vi "ConvertTextBasedCodeToLabVIEW_MakenamesBetter.vi"(11 "ClassesIn":T1[](array[typedef])) -> (3 "ClassesOut":T1[](array[typedef]))   [LabVIEW 2014]
uses:
  <resource>/Framework/Providers/Open_GDS/ClassProviders/Common/String/GDSString_ClassDescriptionType.ctl
  <resource>/Framework/Providers/Open_GDS/ClassProviders/Common/String/GDSString_AccessScopeModifierType.ctl
  <resource>/Framework/Providers/Open_GDS/ClassProviders/Common/String/GDSString_ModifierType.ctl
  <resource>/Framework/Providers/Open_GDS/ClassProviders/Common/String/GDSString_MethodDescriptionType.ctl
  <resource>/Framework/Providers/Open_GDS/ClassProviders/Common/CommonVIs/CommonVIs_AttributeType.ctl
  <resource>/Framework/Providers/Open_GDS/ClassProviders/Common/CommonVIs/CommonVIs_AttributeDataType.ctl
  <resource>/Framework/Providers/Open_GDS/ClassProviders/Common/CommonVIs/CommonVIs_PropertyType.ctl
  <resource>/Framework/Providers/Open_GDS/ClassProviders/Common/String/GDSString_ClassParentType.ctl
  <resource>/Framework/Providers/Open_GDS/ClassProviders/Common/String/GDSString_ClassType.ctl
  <resource>/Framework/Providers/Open_GDS/ClassProviders/Common/String/GDSString_ClassOwnerType.ctl
  <resource>/Framework/Providers/Open_GDS/ClassProviders/Common/CommonVIs/CommonVIs_EnumType.ctl
  <resource>/Framework/Providers/Open_GDS/ClassProviders/Common/CommonVIs/CommonVIs_StructType.ctl
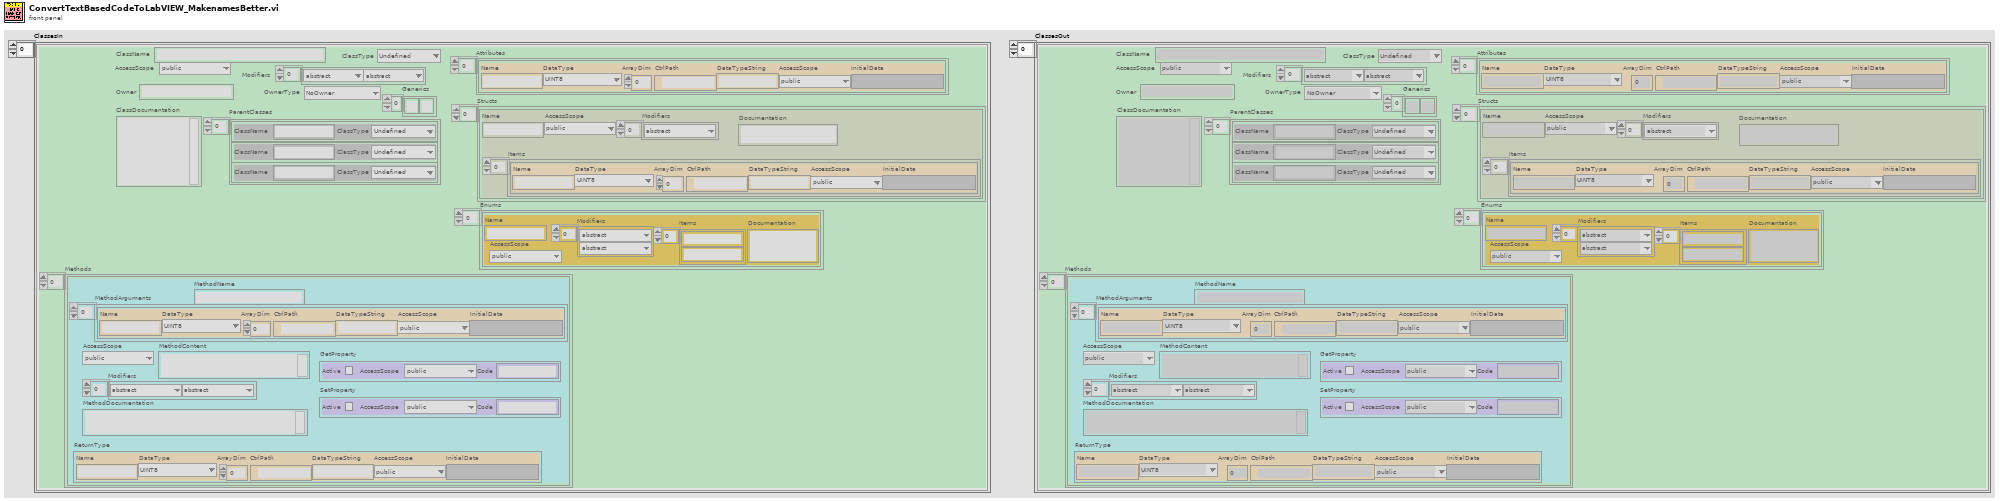
[diagram p1: front panel]
types:
  T1 = typedef "GDSString_ClassDescriptionType.ctl" = cluster{"ClassName":string, "AccessScope":T2, "Modifiers":T3[], "ClassDocumentation":string, "Methods":T4[], "ParentClasses":T8[], "ClassType":T9, "Owner":string, "OwnerType":T10, "Generics":string[], "Attributes":T5[], "Enums":T11[], "Structs":T12[]}
  T2 = typedef "GDSString_AccessScopeModifierType.ctl" = enum16{"public", "private", "protected", "internal"}
  T3 = typedef "GDSString_ModifierType.ctl" = enum16{"abstract", "static", "final", "synchronized", "strictfp", "async", "const", "event", "extern", "new", "native ", "override", "partial", "readonly", "sealed", "unsafe", "virtual", "volatile"}
  T4 = typedef "GDSString_MethodDescriptionType.ctl" = cluster{"ReturnType":T5, "MethodName":string, "AccessScope":T2, "Modifiers":T3[], "MethodDocumentation":string, "MethodContent":string, "MethodArguments":T5[], "GetProperty":T7, "SetProperty":T7}
  T5 = typedef "CommonVIs_AttributeType.ctl" = cluster{"Name":string, "DataType":T6, "ArrayDim":i32, "CtrlPath":path, "DataTypeString":string, "AccessScope":T2, "InitialData":variant}
  T6 = typedef "CommonVIs_AttributeDataType.ctl" = enum16{"UINT8", "INT8", "UINT16", "INT16", "UINT32", "INT32", "UINT64", "INT64", "SGL", "DBL", "EXT", "CSG", "CDB", "CXT", "TimeStamp", "STRING", "PATH", "BOOL", "ENUM", "RefNum", "VIRefNum", "LabVIEW Class", "Cluster", "Variant", "TypeDef", "Waveform", "LabVIEW Object", "Other", "void"}
  T7 = typedef "CommonVIs_PropertyType.ctl" = cluster{"Active":bool, "AccessScope":T2, "Code":string}
  T8 = typedef "GDSString_ClassParentType.ctl" = cluster{"ClassName":string, "ClassType":T9}
  T9 = typedef "GDSString_ClassType.ctl" = enum16{"Undefined", "Class", "Interface"}
  T10 = typedef "GDSString_ClassOwnerType.ctl" = enum16{"NoOwner", "Class", "Package/NameSpace"}
  T11 = typedef "CommonVIs_EnumType.ctl" = cluster{"Name":string, "AccessScope":T2, "Modifiers":T3[], "Items":string[], "Documentation":string}
  T12 = typedef "CommonVIs_StructType.ctl" = cluster{"Name":string, "AccessScope":T2, "Modifiers":T3[], "Items":T5[], "Documentation":string}
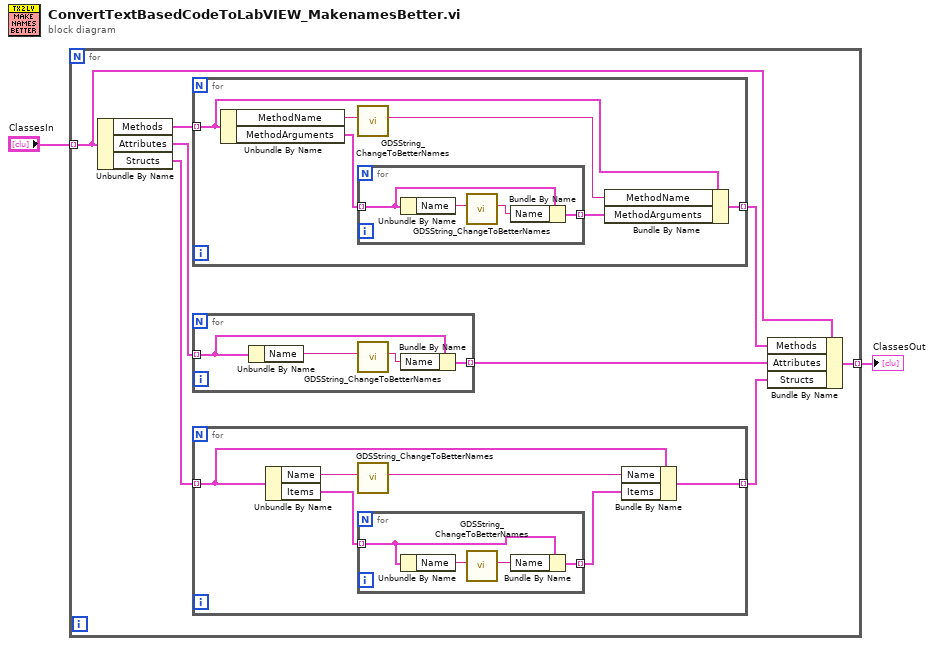
[diagram p0: block diagram]
diagram:
  n1 = for {
    tunnel: "ClassesIn" -> [w8] mode=indexing
    tunnel: [w3] -> w1 mode=indexing
    n2 = Unbundle By Name(w8) -> ("Methods"=w10:T4[], "Attributes"=w9:T5[], "Structs"=w5:T12[])
    n3 = for {
      tunnel: w10 -> [w29] mode=indexing
      tunnel: [w25] -> w7 mode=indexing
      n4 = Unbundle By Name(w29) -> ("MethodName"=w27:string, "MethodArguments"=w30:T5[])
      n5 = call <resource>:"GDSString_ChangeToBetterNames.vi"("NameIn"=w27) -> ("NameOut"=w26:string)  [unwired: 9 in, 1 out]
      n6 = for {
        tunnel: w30 -> [w33] mode=indexing
        tunnel: [w31] -> w28 mode=indexing
        n7 = Unbundle By Name(w33) -> ("Name"=w34:string)
        n8 = call <resource>:"GDSString_ChangeToBetterNames.vi"("NameIn"=w34) -> ("NameOut"=w32:string)  [unwired: 9 in, 1 out]
        n9 = Bundle By Name(cluster=w33, "Name"=w32) -> (w31:T5)
      }
      n10 = Bundle By Name(cluster=w29, "MethodName"=w26, "MethodArguments"=w28) -> (w25:T4)
    }
    n11 = for {
      tunnel: w9 -> [w23] mode=indexing
      tunnel: [w21] -> w6 mode=indexing
      n12 = Unbundle By Name(w23) -> ("Name"=w24:string)
      n13 = call <resource>:"GDSString_ChangeToBetterNames.vi"("NameIn"=w24) -> ("NameOut"=w22:string)  [unwired: 9 in, 1 out]
      n14 = Bundle By Name(cluster=w23, "Name"=w22) -> (w21:T5)
    }
    n15 = for {
      tunnel: w5 -> [w15] mode=indexing
      tunnel: [w11] -> w4 mode=indexing
      n16 = Unbundle By Name(w15) -> ("Name"=w13:string, "Items"=w16:T5[])
      n17 = call <resource>:"GDSString_ChangeToBetterNames.vi"("NameIn"=w13) -> ("NameOut"=w12:string)  [unwired: 9 in, 1 out]
      n18 = for {
        tunnel: w16 -> [w19] mode=indexing
        tunnel: [w17] -> w14 mode=indexing
        n19 = Unbundle By Name(w19) -> ("Name"=w20:string)
        n20 = call <resource>:"GDSString_ChangeToBetterNames.vi"("NameIn"=w20) -> ("NameOut"=w18:string)  [unwired: 9 in, 1 out]
        n21 = Bundle By Name(cluster=w19, "Name"=w18) -> (w17:T5)
      }
      n22 = Bundle By Name(cluster=w15, "Name"=w12, "Items"=w14) -> (w11:T12)
    }
    n23 = Bundle By Name(cluster=w8, "Methods"=w7, "Attributes"=w6, "Structs"=w4) -> (w3:T1)
  }
  "ClassesOut" <- w1
